vi "Request Message.vi"(6 "timeout in ms (-1)":i32=-1, 8 "error in (no error)":errorcluster, 9 "Request Message Data":variant, 10 "Request Message":string, 11 "Process In":refnum<class "Process.lvclass">) -> (0 "error out":errorcluster, 1 "Response Message Data":variant, 2 "Response Message":string, 3 "Process Out":refnum<class "Process.lvclass">, 4 "Timed out?":bool)   [LabVIEW 2020, in "Process.lvclass"]
doc: "Make a syncronous request to the process. The process must respond to the request made using the Response Message.vi method within the configured timeout period to avoid this method from timing out. \nThis method will throw an error if called within the own process loop."
uses:
  Process.lvclass
  C:/git/astemes-triarc-framework/source/Framework/Logging/Logging.lvclass
  Process.lvclass/Process.ctl
  Private/SubVIs/Handle Debug Data.vi
  Logging/Log Debug.vi
  <vilib>/AdvancedString/1D String Array to Delimited String.vi
  <vilib>/Utility/High Resolution Relative Seconds.vi
  Synchronous Request Callback/Synchronous Request Callback.lvclass
  C:/git/astemes-triarc-framework/source/Framework/Callback/Callback.lvclass
  <vilib>/Utility/error.llb/Error Cluster From Error Code.vi
  Public/Read Name.vi
  <vilib>/ErrorRing/Error Ring.xnode
  Callback/Callback.lvclass
  Logging/Logging.lvclass
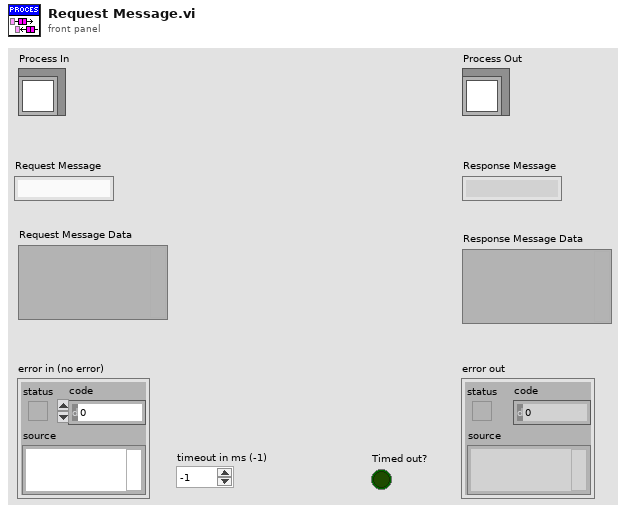
[diagram p1: front panel]
types:
  T1 = typedef "Process.lvclass/API Mode.ctl" = enum16{"Send Message", "Handle Message"}
  T2 = typedef "Process.lvclass/Lifecycle State.ctl" = enum16{"Uninitialized", "Initialized", "Started", "Running", "Stopped", "Finished"}
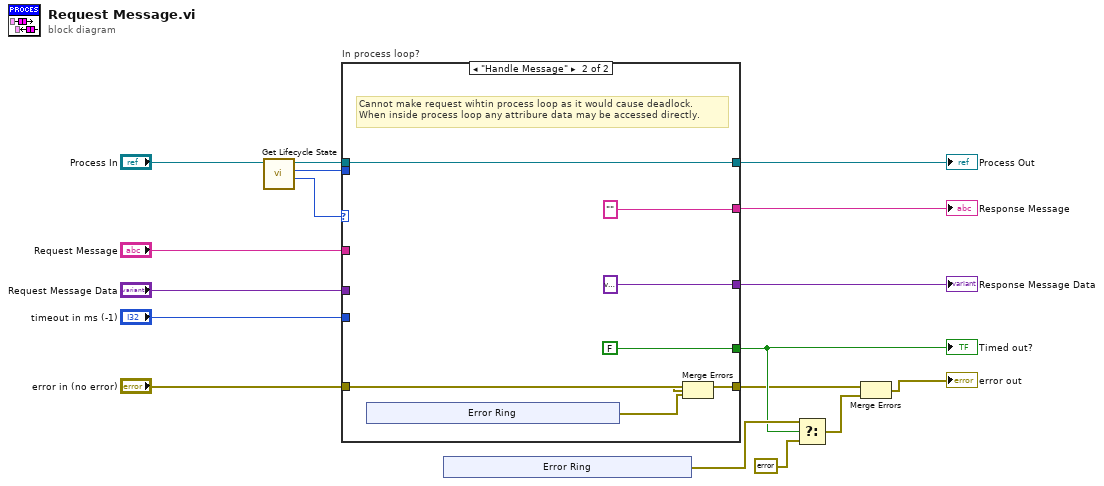
[diagram p0: block diagram]
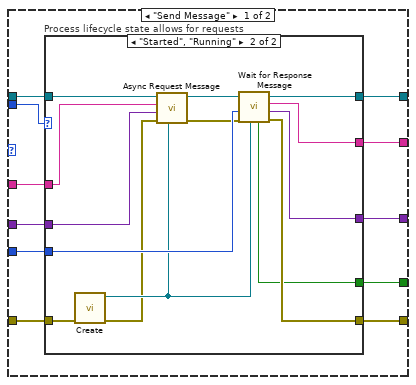
[diagram p2: hidden frame]
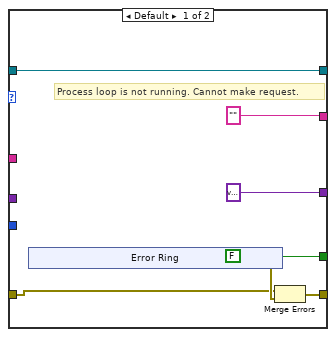
[diagram p3: hidden frame]
diagram:
  n1 = call "Get Lifecycle State.vi"("Process In"="Process In") -> ("API Mode"=w3:T1, "Lifecycle State"=w2:T2, "Process Out"=w4:refnum<class "Process.lvclass">)  [unwired: 7 in, 1 out]
  n2 = case "In process loop?" shown="\"Handle Message\"" w3 {
    tunnel: "Request Message" -> [w28 _]
    tunnel: "Request Message Data" -> [w27 _]
    tunnel: [w26 w60] -> w15
    tunnel: "timeout in ms (-1)" -> [w25 _]
    tunnel: [w24 w55] -> w10
    tunnel: w4 -> [w23 w60]
    tunnel: "error in (no error)" -> [w22 w56]
    tunnel: [w21 FALSE ("timed out?")] -> w11
    tunnel: [w20 "" ("Message")] -> w8
    tunnel: [w19 variant ("Message Data")] -> w9
    tunnel: w2 -> [w18 _]
    frame "Send Message" {
      n3 = case "Process lifecycle state allows for requests" shown="\"Started\", \"Running\"" w18 {
        tunnel: w28 -> [_ w44]
        tunnel: w27 -> [_ w43]
        tunnel: [w29 w49] -> w26
        tunnel: w25 -> [_ w48]
        tunnel: [w33 w51] -> w24
        tunnel: w23 -> [w29 w50]
        tunnel: w22 -> [w34 w40]
        tunnel: [FALSE ("timed out?") w47] -> w21
        tunnel: ["" ("Message") w53] -> w20
        tunnel: [variant ("Message Data") w52] -> w19
        frame Default {
          # "Process loop is not running. Cannot make request."
          n4 = xnode "Error Ring"() -> ("error out"=w35:errorcluster)
          n5 = Merge Errors(w34, w35) -> (w33:errorcluster)
        }
        frame "Started", "Running" {
          n6 = call "Create.vi"("error in (no error)"=w40) -> ("error out"=w41:errorcluster, "Synchronous Request Callback Out"=w42:refnum<class "Synchronous Request Callback.lvclass">)  [unwired: 9 in]
          n7 = call "Async Request Message.vi"("Callback"=w42, "error in (no error)"=w41, "Request Message Data"=w43, "Request Message"=w44, "Process In"=w50) -> ("error out"=w46:errorcluster, "Process Out"=w45:refnum<class "Process.lvclass">)  [unwired: 3 in]
          n8 = call "Wait for Response Message.vi"("Synchronous Request Callback"=w42, "error in (no error)"=w46, "timeout in ms"=w48, "Process In"=w45) -> ("error out"=w51:errorcluster, "Message Data"=w52:variant, "Message"=w53:string, "Process Out"=w49:refnum<class "Process.lvclass">, "timed out?"=w47:bool)  [unwired: 3 in]
        }
      }
    }
    frame "Handle Message" {
      # "Cannot make request wihtin process loop as it would cause deadlock.\nWhen inside process loop any attribure data may be accessed directly."
      n9 = xnode "Error Ring"() -> ("error out"=w54:errorcluster)
      n10 = Merge Errors(w56, w54) -> (w55:errorcluster)
    }
  }
  "Process Out" <- w15
  "Response Message" <- w8
  "Response Message Data" <- w9
  "Timed out?" <- w11
  n11 = xnode "Error Ring"() -> ("error out"=w12:errorcluster)
  n12 = Select(t=w12, s=w11, f=errorcluster {"status"=FALSE, "code"=0, "source"=""}) -> (s? t:f=w7:errorcluster)
  n13 = Merge Errors(w10, w7) -> (→"error out":errorcluster)
